vi "HFRR ADV v02.vi"() -> ()   [LabVIEW 2025] (continued)
            n3115 = local read "S 84"() -> (w4160:string)
            n3116 = local read "S 103"() -> (w4145:string)
            n3117 = local read "S 104"() -> (w4144:string)
            n3118 = property on="ENTER THE NEW PASSWORD" class="Str"("Caption.Text"=w4157) -> ()  [unwired: 2 in, 2 out]
            n3119 = property on="Password" class="Str"("Caption.Text"=w4159) -> ()  [unwired: 2 in, 2 out]
            n3120 = property on="ENTER CURRENT PASSWORD" class="Str"("Caption.Text"=w4158) -> ()  [unwired: 2 in, 2 out]
            n3121 = property on="EDIT" class="Bool (strict)"("Boolean Text.Text"=w4156) -> ()  [unwired: 2 in, 2 out]
            n3122 = property on="SAVE" class="Bool (strict)"("Boolean Text.Text"=w4160) -> ()  [unwired: 2 in, 2 out]
            n3123 = Build Array(w4145, w4144) -> (w4143:string[])
            n3124 = property on="Heater Button" class="Bool (strict)"("Strings [4]"=w4143) -> ()  [unwired: 2 in, 2 out]
            n3125 = property on="CH-HUMIDITY WET" class="DigNum (strict)"("Caption.Size to Text?"=w4146) -> ()  [unwired: 2 in, 2 out]
            n3126 = property on="CH-HUMIDITY DRY" class="DigNum (strict)"("Caption.Size to Text?"=w4146) -> ()  [unwired: 2 in, 2 out]
            n3127 = property on="CH-POWER -" class="DigNum (strict)"("Caption.Size to Text?"=w4146) -> ()  [unwired: 2 in, 2 out]
            n3128 = property on="CH-HEATER" class="DigNum (strict)"("Caption.Size to Text?"=w4146) -> ()  [unwired: 2 in, 2 out]
            n3129 = property on="CH-POWER +" class="DigNum (strict)"("Caption.Size to Text?"=w4146) -> ()  [unwired: 2 in, 2 out]
            n3130 = local read "S 92"() -> (w4155:string)
            n3131 = local read "S 93"() -> (w4154:string)
            n3132 = local read "S 105"() -> (w4141:string)
            n3133 = local read "S 106"() -> (w4140:string)
            n3134 = Build Array(w4155, w4154) -> ()  [unwired: 1 out]
            n3135 = Build Array(w4141, w4140) -> (w4142:string[])
            n3136 = local read "S 95"() -> (w4152:string)
            n3137 = local read "S 94"() -> (w4153:string)
            n3138 = local read "bs"() -> (w4168:string)
            n3139 = local read "as"() -> (w4169:string)
            n3140 = property on="Humidity" class="Bool (strict)"("Strings [4]"=w4142) -> ()  [unwired: 2 in, 2 out]
            n3141 = Concatenate Strings(w4168, "\r", w4169) -> ()  [unwired: 1 out]
            n3142 = property on="STROKE GAIN :" class="DigNum (strict)"("Caption.Text"=w4152) -> ()  [unwired: 2 in, 2 out]
            n3143 = property on="DISPLACEMENT :" class="DigNum (strict)"("Caption.Text"=w4153) -> ()  [unwired: 2 in, 2 out]
            n3144 = property on="Rh After" class="DigNum (strict)"("Caption.Size to Text?"=TRUE ("Caption.Size to Text")) -> ()  [unwired: 2 in, 2 out]
            n3145 = local read "S 48"() -> (w4192:string)
            n3146 = local read "S 50"() -> (w4190:string)
            n3147 = local read "S 51"() -> (w4189:string)
            n3148 = local read "S 49"() -> (w4191:string)
            n3149 = local read "S 52"() -> (w4188:string)
            n3150 = local read "as"() -> (w4173:string)
            n3151 = local read "bs"() -> (w4174:string)
            n3152 = local read "S 56"() -> (w4187:string)
            n3153 = local read "S 57"() -> (w4186:string)
            n3154 = local read "S 58"() -> (w4185:string)
            n3155 = local read "S 59"() -> (w4184:string)
            n3156 = property on="OPEN" class="Bool (strict)"("Boolean Text.Text"=w4188) -> ()  [unwired: 2 in, 2 out]
            n3157 = property on="OPEN 1" class="Bool (strict)"("Boolean Text.Text"=w4192) -> ()  [unwired: 2 in, 2 out]
            n3158 = property on="OPEN 2" class="Bool (strict)"("Boolean Text.Text"=w4191) -> ()  [unwired: 2 in, 2 out]
            n3159 = property on="OPEN 3" class="Bool (strict)"("Boolean Text.Text"=w4190) -> ()  [unwired: 2 in, 2 out]
            n3160 = property on="OPEN 4" class="Bool (strict)"("Boolean Text.Text"=w4189) -> ()  [unwired: 2 in, 2 out]
            n3161 = Concatenate Strings(w4174, "\r", w4173) -> ()  [unwired: 1 out]
            n3162 = local read "S 102"() -> (w4147:string)
            n3163 = property on="КОФ1" class="DigNum (strict)"("Caption.Text"=w4187) -> ()  [unwired: 2 in, 2 out]
            n3164 = local read "S 98"() -> (w4151:string)
            n3165 = local read "S 99"() -> (w4150:string)
            n3166 = local read "S 100"() -> (w4149:string)
            n3167 = local read "S 101"() -> (w4148:string)
            n3168 = property on="КОФ2" class="DigNum (strict)"("Caption.Text"=w4186) -> ()  [unwired: 2 in, 2 out]
            n3169 = property on="КОФ3" class="DigNum (strict)"("Caption.Text"=w4185) -> ()  [unwired: 2 in, 2 out]
            n3170 = property on="КОФ4" class="DigNum (strict)"("Caption.Text"=w4184) -> ()  [unwired: 2 in, 2 out]
            n3171 = local read "bs"() -> (w4172:string)
            n3172 = local read "as"() -> (w4171:string)
            n3173 = property on="CH-POWER +" class="DigNum (strict)"("Caption.Text"=w4151) -> ()  [unwired: 2 in, 2 out]
            n3174 = property on="CH-POWER -" class="DigNum (strict)"("Caption.Text"=w4150) -> ()  [unwired: 2 in, 2 out]
            n3175 = property on="CH-HEATER" class="DigNum (strict)"("Caption.Text"=w4149) -> ()  [unwired: 2 in, 2 out]
            n3176 = property on="CH-HUMIDITY DRY" class="DigNum (strict)"("Caption.Text"=w4148) -> ()  [unwired: 2 in, 2 out]
            n3177 = property on="CH-HUMIDITY WET" class="DigNum (strict)"("Caption.Text"=w4147) -> ()  [unwired: 2 in, 2 out]
            n3178 = local read "S 60"() -> (w4183:string)
            n3179 = local read "S 54"() -> (w4193:string)
            n3180 = Concatenate Strings(w4172, "\r", w4171) -> ()  [unwired: 1 out]
            n3181 = Concatenate Strings(w4193, w4183) -> ()  [unwired: 1 out]
            n3182 = local read "S 77"() -> (→"String 43":string)
            n3183 = local read "S 76"() -> (w4166:string)
            n3184 = local read "S 78"() -> (w4165:string)
            n3185 = local read "S 71"() -> (w4177:string)
            n3186 = local read "S 66"() -> (w4182:string)
            n3187 = local read "S 67"() -> (w4181:string)
            n3188 = local read "S 68"() -> (w4180:string)
            n3189 = local read "S 69"() -> (w4179:string)
            n3190 = local read "S 70"() -> (w4178:string)
            n3191 = property on="AIR TEMP" class="DigNum (strict)"("Caption.Text"=w4165) -> ()  [unwired: 2 in, 2 out]
            n3192 = property on="Set Strk" class="DigNum (strict)"("Caption.Text"=w4166) -> ()  [unwired: 2 in, 2 out]
            n3193 = property on="FRIC. FORCE :" class="DigNum (strict)"("Caption.Text"=w4182) -> ()  [unwired: 2 in, 2 out]
            n3194 = property on="TEMPERATURE :" class="DigNum (strict)"("Caption.Text"=w4181) -> ()  [unwired: 2 in, 2 out]
            n3195 = property on="SPEED OUT:" class="DigNum (strict)"("Caption.Text"=w4180) -> ()  [unwired: 2 in, 2 out]
            n3196 = property on="AIR TEMPERATURE :" class="DigNum (strict)"("Caption.Text"=w4179) -> ()  [unwired: 2 in, 2 out]
            n3197 = property on="HUMIDITY:" class="DigNum (strict)"("Caption.Text"=w4178) -> ()  [unwired: 2 in, 2 out]
            n3198 = property on="EDIT" class="Bool (strict)"("Boolean Text.Text"=w4177) -> ()  [unwired: 2 in, 2 out]
            n3199 = local read "S 79"() -> (w4164:string)
          }
          frame #2 {
          }
        }
        n3200 = local write "Lan flag"(10.0 ("Lan flag")) -> ()
      }
      frame Enabled {
      }
    }
    n3201 = Wait (ms)(milliseconds to wait=u32 2000) -> ()  [unwired: 1 out]
    n3202 = local read "Quit"() -> (w3967:bool)
  }
  n3203 = disable-structure shown="Disabled" {
    frame Disabled {
      n3204 = while {
        tunnel: [w4195] -> _
        i -> [w4195]
        stop <- w4194 continue-if-true
        n3205 = Wait (ms)(milliseconds to wait=u32 50) -> ()  [unwired: 1 out]
        n3206 = stacked-sequence {
          frame #0 {
            # "Controls Text color"
            # "Controls BG color"
            n3207 = property on="FILE" class="Str"("Text.Text Colors:Text Color"="SC  Text") -> ()  [unwired: 2 in, 2 out]
            n3208 = property on="Fuel Discription :" class="Str"("Text.Text Colors:Text Color"="SC  Text") -> ()  [unwired: 2 in, 2 out]
            n3209 = property on="tested by" class="Str"("Text.Text Colors:Text Color"="SC  Text") -> ()  [unwired: 2 in, 2 out]
            n3210 = property on="Remarks :" class="Str"("Text.Text Colors:Text Color"="SC  Text") -> ()  [unwired: 2 in, 2 out]
            n3211 = property class="DigNum (strict)"("Numeric Text.Text Colors:BG Color"="NC BG") -> ()  [unwired: 2 in, 2 out]
            n3212 = property class="DigNum (strict)"("Numeric Text.Text Colors:BG Color"="NC BG") -> ()  [unwired: 2 in, 2 out]
            n3213 = property class="DigNum (strict)"("Numeric Text.Text Colors:BG Color"="NC BG") -> ()  [unwired: 2 in, 2 out]
            n3214 = property class="DigNum (strict)"("Numeric Text.Text Colors:BG Color"="NC BG") -> ()  [unwired: 2 in, 2 out]
            n3215 = property class="DigNum (strict)"("Numeric Text.Text Colors:BG Color"="NC BG") -> ()  [unwired: 2 in, 2 out]
            n3216 = property class="DigNum (strict)"("Numeric Text.Text Colors:BG Color"="NC BG") -> ()  [unwired: 2 in, 2 out]
            n3217 = property class="DigNum (strict)"("Numeric Text.Text Colors:BG Color"="NC BG") -> ()  [unwired: 2 in, 2 out]
            n3218 = property class="DigNum (strict)"("Numeric Text.Text Colors:BG Color"="NC BG") -> ()  [unwired: 2 in, 2 out]
            n3219 = property class="DigNum (strict)"("Numeric Text.Text Colors:BG Color"="NC BG") -> ()  [unwired: 2 in, 2 out]
            n3220 = property class="DigNum (strict)"("Numeric Text.Text Colors:BG Color"="NC BG") -> ()  [unwired: 2 in, 2 out]
            n3221 = property class="DigNum (strict)"("Numeric Text.Text Colors:BG Color"="NC BG") -> ()  [unwired: 2 in, 2 out]
            n3222 = property class="DigNum (strict)"("Numeric Text.Text Colors:BG Color"="NC BG") -> ()  [unwired: 2 in, 2 out]
            n3223 = property on="FILE" class="Str"("Text.Text Colors:BG Color"="SC BG 3") -> ()  [unwired: 2 in, 2 out]
            n3224 = property on="Fuel Discription :" class="Str"("Text.Text Colors:BG Color"="SC BG 3") -> ()  [unwired: 2 in, 2 out]
            n3225 = property on="tested by" class="Str"("Text.Text Colors:BG Color"="SC BG 3") -> ()  [unwired: 2 in, 2 out]
            n3226 = property on="Remarks :" class="Str"("Text.Text Colors:BG Color"="SC BG 3") -> ()  [unwired: 2 in, 2 out]
            n3227 = property class="DigNum (strict)"("Numeric Text.Text Colors:Text Color"="NC Text") -> ()  [unwired: 2 in, 2 out]
            n3228 = property class="DigNum (strict)"("Numeric Text.Text Colors:Text Color"="NC Text") -> ()  [unwired: 2 in, 2 out]
            n3229 = property class="DigNum (strict)"("Numeric Text.Text Colors:Text Color"="NC Text") -> ()  [unwired: 2 in, 2 out]
            n3230 = property class="DigNum (strict)"("Numeric Text.Text Colors:Text Color"="NC Text") -> ()  [unwired: 2 in, 2 out]
            n3231 = property class="DigNum (strict)"("Numeric Text.Text Colors:Text Color"="NC Text") -> ()  [unwired: 2 in, 2 out]
            n3232 = property class="DigNum (strict)"("Numeric Text.Text Colors:Text Color"="NC Text") -> ()  [unwired: 2 in, 2 out]
            n3233 = property class="DigNum (strict)"("Numeric Text.Text Colors:Text Color"="NC Text") -> ()  [unwired: 2 in, 2 out]
            n3234 = property class="DigNum (strict)"("Numeric Text.Text Colors:Text Color"="NC Text") -> ()  [unwired: 2 in, 2 out]
            n3235 = property class="DigNum (strict)"("Numeric Text.Text Colors:Text Color"="NC Text") -> ()  [unwired: 2 in, 2 out]
            n3236 = property class="DigNum (strict)"("Numeric Text.Text Colors:Text Color"="NC Text") -> ()  [unwired: 2 in, 2 out]
            n3237 = property class="DigNum (strict)"("Numeric Text.Text Colors:Text Color"="NC Text") -> ()  [unwired: 2 in, 2 out]
            n3238 = property class="DigNum (strict)"("Numeric Text.Text Colors:Text Color"="NC Text") -> ()  [unwired: 2 in, 2 out]
            n3239 = property class="DigNum (strict)"("Numeric Text.Text Colors:Text Color"="NI Text  2") -> ()  [unwired: 2 in, 2 out]
            n3240 = property class="DigNum (strict)"("Numeric Text.Text Colors:Text Color"="NI Text  2") -> ()  [unwired: 2 in, 2 out]
            n3241 = property class="DigNum (strict)"("Numeric Text.Text Colors:Text Color"="NI Text  2") -> ()  [unwired: 2 in, 2 out]
            n3242 = property class="DigNum (strict)"("Numeric Text.Text Colors:Text Color"="NI Text  2") -> ()  [unwired: 2 in, 2 out]
            n3243 = property class="DigNum (strict)"("Numeric Text.Text Colors:Text Color"="NI Text  2") -> ()  [unwired: 2 in, 2 out]
            n3244 = property class="DigNum (strict)"("Numeric Text.Text Colors:Text Color"="NI Text  2") -> ()  [unwired: 2 in, 2 out]
            n3245 = property class="DigNum (strict)"("Numeric Text.Text Colors:Text Color"="NI Text  2") -> ()  [unwired: 2 in, 2 out]
            n3246 = property class="DigNum (strict)"("Numeric Text.Text Colors:Text Color"="NI Text  2") -> ()  [unwired: 2 in, 2 out]
            n3247 = property class="DigNum (strict)"("Numeric Text.Text Colors:Text Color"="NI Text  2") -> ()  [unwired: 2 in, 2 out]
            n3248 = property class="DigNum (strict)"("Numeric Text.Text Colors:Text Color"="NI Text  2") -> ()  [unwired: 2 in, 2 out]
            n3249 = property class="DigNum (strict)"("Numeric Text.Text Colors:Text Color"="NI Text  2") -> ()  [unwired: 2 in, 2 out]
            n3250 = property class="DigNum (strict)"("Numeric Text.Text Colors:Text Color"="NI Text  2") -> ()  [unwired: 2 in, 2 out]
            n3251 = property class="DigNum (strict)"("Numeric Text.Text Colors:Text Color"="NI Text  2") -> ()  [unwired: 2 in, 2 out]
            n3252 = property class="DigNum (strict)"("Numeric Text.Text Colors:Text Color"="NI Text  2") -> ()  [unwired: 2 in, 2 out]
            n3253 = property class="DigNum (strict)"("Numeric Text.Text Colors:Text Color"="NI Text  2") -> ()  [unwired: 2 in, 2 out]
            n3254 = property on="Coefficient Of Friction" class="XYGraph (strict)"("Plot Area:Colors:FG Color"="GFG  2", "Plot Area:Colors:BG Color"="GBG   2") -> ()  [unwired: 2 in, 2 out]
            n3255 = property on="Humidity ( %RH )" class="XYGraph (strict)"("Plot Area:Colors:FG Color"="GFG  2", "Plot Area:Colors:BG Color"="GBG   2") -> ()  [unwired: 2 in, 2 out]
            n3256 = property on="Air Temperature  ( °C )" class="XYGraph (strict)"("Plot Area:Colors:FG Color"="GFG  2", "Plot Area:Colors:BG Color"="GBG   2") -> ()  [unwired: 2 in, 2 out]
            n3257 = property on="Sample Temperature ( °C )" class="XYGraph (strict)"("Plot Area:Colors:FG Color"="GFG  2", "Plot Area:Colors:BG Color"="GBG   2") -> ()  [unwired: 2 in, 2 out]
            n3258 = property class="DigNum (strict)"("Numeric Text.Text Colors:BG Color"="NI BG 2") -> ()  [unwired: 2 in, 2 out]
            n3259 = property class="DigNum (strict)"("Numeric Text.Text Colors:BG Color"="NI BG 2") -> ()  [unwired: 2 in, 2 out]
            n3260 = property class="DigNum (strict)"("Numeric Text.Text Colors:BG Color"="NI BG 2") -> ()  [unwired: 2 in, 2 out]
            n3261 = property class="DigNum (strict)"("Numeric Text.Text Colors:BG Color"="NI BG 2") -> ()  [unwired: 2 in, 2 out]
            n3262 = property class="DigNum (strict)"("Numeric Text.Text Colors:BG Color"="NI BG 2") -> ()  [unwired: 2 in, 2 out]
            n3263 = property class="DigNum (strict)"("Numeric Text.Text Colors:BG Color"="NI BG 2") -> ()  [unwired: 2 in, 2 out]
            n3264 = property class="DigNum (strict)"("Numeric Text.Text Colors:BG Color"="NI BG 2") -> ()  [unwired: 2 in, 2 out]
            n3265 = property class="DigNum (strict)"("Numeric Text.Text Colors:BG Color"="NI BG 2") -> ()  [unwired: 2 in, 2 out]
            n3266 = property class="DigNum (strict)"("Numeric Text.Text Colors:BG Color"="NI BG 2") -> ()  [unwired: 2 in, 2 out]
            n3267 = property class="DigNum (strict)"("Numeric Text.Text Colors:BG Color"="NI BG 2") -> ()  [unwired: 2 in, 2 out]
            n3268 = property class="DigNum (strict)"("Numeric Text.Text Colors:BG Color"="NI BG 2") -> ()  [unwired: 2 in, 2 out]
            n3269 = property class="DigNum (strict)"("Numeric Text.Text Colors:BG Color"="NI BG 2") -> ()  [unwired: 2 in, 2 out]
            n3270 = property class="DigNum (strict)"("Numeric Text.Text Colors:BG Color"="NI BG 2") -> ()  [unwired: 2 in, 2 out]
            n3271 = property class="DigNum (strict)"("Numeric Text.Text Colors:BG Color"="NI BG 2") -> ()  [unwired: 2 in, 2 out]
            n3272 = property class="DigNum (strict)"("Numeric Text.Text Colors:BG Color"="NI BG 2") -> ()  [unwired: 2 in, 2 out]
            n3273 = property class="Bool"("Colors [4]"="Boolean BC T & BG") -> ()  [unwired: 2 in, 2 out]
            n3274 = property on="Save & Continue" class="Bool (strict)"("Colors [4]"="Boolean BC T & BG") -> ()  [unwired: 2 in, 2 out]
            n3275 = property on="Heater Button" class="Bool (strict)"("Colors [4]"="Boolean BC T & BG") -> ()  [unwired: 2 in, 2 out]
            n3276 = property class="Bool"("Colors [4]"="Boolean BC T & BG") -> ()  [unwired: 2 in, 2 out]
            n3277 = property on="Humidity" class="Bool (strict)"("Colors [4]"="Boolean BC T & BG") -> ()  [unwired: 2 in, 2 out]
            n3278 = property class="Bool (strict)"("Colors [4]"="Boolean BC T & BG") -> ()  [unwired: 2 in, 2 out]
            n3279 = property on="RUN" class="Bool (strict)"("Colors [4]"="Boolean BC T & BG") -> ()  [unwired: 2 in, 2 out]
            n3280 = property on="trip1 8" class="Bool (strict)"("Colors [4]"="Boolean BC T & BG") -> ()  [unwired: 2 in, 2 out]
            n3281 = property class="Bool"("Colors [4]"="Boolean BC T & BG") -> ()  [unwired: 2 in, 2 out]
            n3282 = property class="Bool (strict)"("Colors [4]"="Boolean BC T & BG") -> ()  [unwired: 2 in, 2 out]
            n3283 = property on="OPEN 1" class="Bool (strict)"("Colors [4]"="Boolean BC T & BG 2") -> ()  [unwired: 2 in, 2 out]
            n3284 = property on="OPEN 2" class="Bool (strict)"("Colors [4]"="Boolean BC T & BG 2") -> ()  [unwired: 2 in, 2 out]
            n3285 = property on="OPEN 3" class="Bool (strict)"("Colors [4]"="Boolean BC T & BG 2") -> ()  [unwired: 2 in, 2 out]
            n3286 = property on="OPEN 4" class="Bool (strict)"("Colors [4]"="Boolean BC T & BG 2") -> ()  [unwired: 2 in, 2 out]
            n3287 = property on="OPEN" class="Bool (strict)"("Colors [4]"="Boolean BC T & BG 2") -> ()  [unwired: 2 in, 2 out]
            n3288 = property on="rstv2" class="Bool"("Colors [4]"="Boolean BC T & BG 2") -> ()  [unwired: 2 in, 2 out]
            n3289 = property on="RST CP" class="Bool"("Colors [4]"="Boolean BC T & BG 2") -> ()  [unwired: 2 in, 2 out]
            n3290 = property on="RSTV1 3" class="Bool"("Colors [4]"="Boolean BC T & BG 2") -> ()  [unwired: 2 in, 2 out]
            n3291 = property on="RSTV1 2" class="Bool"("Colors [4]"="Boolean BC T & BG 2") -> ()  [unwired: 2 in, 2 out]
          }
          frame #1 {
          }
        }
        n3292 = local read "Quit"() -> (w4194:bool)
      }
    }
    frame Enabled {
    }
  }
  n3293 = while {
    shift-right: [w4212] -> _
    shift-left: _ -> [w4213]
    shift-right: [w4210] -> _
    shift-left: T14 {"Read Heave and Surge"="", "Bytes at Heave Port"=0.0, "Heave and Surge COM Port:"="COM9", "Com Port 2"="COM7", "Residual Due"="", "Heave COM Status 2"=TRUE, "Heave COM Status"=TRUE, "Port 2"=TRUE, "Sway PPR"=6400.0, "Surge PPR"=6400.0, "Heave PPR"=6400.0, "Sway Pitch"=2.0, "Surge Pitch"=3.0, "Heave Pitch"=4.0, "Sway Pulses/mm"=320.0, "Surge Pulses/mm"=1600.0, "Heave Pulses/mm"=1600.0, "inner loop"=0.0, "Read Heave and Surge 2"="", "String 36"="", "Write S"=FALSE, "WriteCC1"=[""], "Heave COM Loop"=0, "LastCom"="", "EXIT"=FALSE, "Error Heave"={"status"=TRUE, "code"=-1073807343, "source"=""}} -> [w4209]
    shift-right: [w4207] -> _
    shift-left: enum16{"init", "MAIN", "Panel Close"}."init" -> [w4208]
    stop <- w4211 stop-if-true
    n3294 = case shown="\"init\"" w4208 {
      tunnel: w4213 -> [w4227 w4242 w4312 w4314]
      tunnel: [w4221 w4260 w4312 w4314] -> w4212
      tunnel: [_ _ TRUE _] -> w4211
      tunnel: [w4217 w4257 w4310 w4313] -> w4210
      tunnel: w4209 -> [w4224 w4241 w4310 w4313]
      tunnel: [enum16{"init", "MAIN", "Panel Close"}."MAIN" w4235 _ _] -> w4207
      frame "init" {
        n3295 = Bundle By Name(cluster=w4224, "Heave and Surge COM Port:"="C3 :") -> (w4223:T14)
        n3296 = call "Instrument fgv.vi"("Enum"=T24."INIT", "error in (no error) 2"=w4227, "INPUT"=w4223) -> ("error"=w4225:errorcluster, "output"=w4220:T14)  [unwired: 6 in, 1 out]
        n3297 = case shown="No Error" w4225 {
          selector: w4225 -> [w4229 _]
          tunnel: [w4229 w4233] -> w4221
          tunnel: w4220 -> [w4228 w4231]
          tunnel: [w4228 w4230] -> w4218
          frame No Error {
          }
          frame Error {
            n3298 = call "Instrument fgv.vi"("Enum"=T24."ERROR INIT", "INPUT"=w4231) -> ("error"=w4234:errorcluster, "output"=w4230:T14)  [unwired: 7 in, 1 out]
            n3299 = call <vilib>:"Clear Errors.vi"("error in (no error)"=w4234) -> ("error out"=w4233:errorcluster)  [unwired: 5 in, 1 out]
          }
        }
        n3300 = local read "LastCom"() -> (w4216:string)
        n3301 = Unbundle By Name(w4218) -> ("Heave COM Status 2"=→"COM Status" →"Instrument Status":bool, "Error Heave"=→"Error":errorcluster)  [unwired: 1 out]
        n3302 = Bundle By Name(cluster=w4218, "LastCom"=w4216) -> (w4217:T14)
      }
      frame "MAIN" {
        n3303 = Unbundle By Name(w4241) -> ("Com Port 2"=w4262:refnum<visa-resource-name>)
        n3304 = local write "Com Port 4"(w4262) -> ()
        n3305 = local read "C3 :"() -> (w4239:refnum<visa-resource-name>)
        n3306 = Divide(x="Heave PPR", y="Heave Pitch") -> (x/y=→"Heave Pulses/mm":dbl)
        n3307 = Bundle By Name(cluster=w4241, "Heave and Surge COM Port:"=w4239) -> (w4240:T14)
        n3308 = Equal?(x=w4262, y=w4239) -> (x = y?=w4261:bool)
        n3309 = Divide(x="Sway PPR", y="Sway Pitch") -> (x/y=→"Sway Pulses/mm":dbl)
        n3310 = case shown="False" w4261 {
          tunnel: [w4266 w4283] -> w4260
          tunnel: w4242 -> [w4267 w4289]
          tunnel: w4240 -> [w4265 w4287]
          tunnel: [w4264 w4282] -> w4257
          frame False {
            n3311 = call <vilib>:"Clear Errors.vi"("error in (no error)"=w4267) -> ("error out"=w4263:errorcluster)  [unwired: 5 in, 1 out]
            n3312 = call "Instrument fgv.vi"("Enum"=T24."ERROR INIT", "error in (no error) 2"=w4263, "INPUT"=w4265) -> ("error"=w4269:errorcluster, "output"=w4264:T14)  [unwired: 6 in, 1 out]
            n3313 = call <vilib>:"Clear Errors.vi"("error in (no error)"=w4269) -> ("error out"=w4266:errorcluster)  [unwired: 5 in, 1 out]
          }
          frame True {
            n3314 = call "Instrument fgv.vi"("Enum"=T24."READ", "error in (no error) 2"=w4289, "INPUT"=w4287) -> ("error"=w4288:errorcluster, "output"=w4279:T14)  [unwired: 6 in, 1 out]
            n3315 = Bundle By Name(cluster=w4279, "String 36"="String 11") -> (w4278:T14)
            n3316 = case shown="True" "Write S" {
              selector: "Write S" -> [_ w4309]
              tunnel: w4288 -> [w4302 w4308]
              tunnel: [w4302 w4307] -> w4275
              tunnel: w4278 -> [w4301 w4304]
              tunnel: [w4301 w4303] -> w4274
              frame False {
              }
              frame True {
                n3317 = Not(x=w4309) -> (.not. x?=w4305:bool)
                n3318 = local write "Write S"(w4305) -> ()
                n3319 = call "Instrument fgv.vi"("Enum"=T24."MANUAL WRITE", "error in (no error) 2"=w4308, "INPUT"=w4304) -> ("error"=w4307:errorcluster, "output"=w4303:T14)  [unwired: 6 in, 1 out]
              }
            }
            n3320 = Array Size(array="WriteHumidity") -> (size(s)=w4272:i32)
            n3321 = Greater Than 0?(x=w4272) -> (x > 0?=w4270:bool)
            n3322 = call "Instrument fgv.vi"("Enum"=T24."WRITE", "error in (no error) 2"=w4275, "WriteCC1"="WriteHumidity", "INPUT"=w4274) -> ("error"=w4285:errorcluster, "WriteCC1 2"=w4273:string[], "output"=w4284:T14)  [unwired: 5 in]
            n3323 = case shown="True" w4270 {
              tunnel: w4273 -> [_ w4291]
              frame False {
              }
              frame True {
                n3324 = local write "WriteHumidity"(w4291) -> ()
              }
            }
            n3325 = case shown="Error" w4285 {
              selector: w4285 -> [w4292 w4295]
              tunnel: w4284 -> [w4293 w4300]
              tunnel: [w4293 w4299] -> w4282
              tunnel: [w4292 w4297] -> w4283
              frame No Error {
              }
              frame Error {
                n3326 = call <vilib>:"Clear Errors.vi"("error in (no error)"=w4295) -> ("error out"=w4294:errorcluster)  [unwired: 5 in, 1 out]
                n3327 = call "Instrument fgv.vi"("Enum"=T24."ERROR INIT", "error in (no error) 2"=w4294, "INPUT"=w4300) -> ("error"=w4298:errorcluster, "output"=w4299:T14)  [unwired: 6 in, 1 out]
                n3328 = call <vilib>:"Clear Errors.vi"("error in (no error)"=w4298) -> ("error out"=w4297:errorcluster)  [unwired: 5 in, 1 out]
              }
            }
            n3329 = Unbundle By Name(w4282) -> ("LastCom"=→"LastCom":string, "Read Heave and Surge"=→"Read Humidity":string)
          }
        }
        n3330 = Divide(x="Surge PPR", y="Surge Pitch") -> (x/y=→"Surge Pulses/mm":dbl)
        n3331 = Unbundle By Name(w4257) -> ("Heave COM Status 2"=w4259:bool, "Heave COM Status"=w4258:bool, "Error Heave"=w4255:errorcluster, "Bytes at Heave Port"=→"Bytes at Humidity Port":dbl)
        n3332 = Unbundle By Name(w4255) -> ("status"=→"Humidity Port":bool)
        n3333 = Not(x=w4258) -> (.not. x?=w4243:bool)
        n3334 = local write "Error"(w4255) -> ()
        n3335 = Not(x=w4259) -> (.not. x?=w4244:bool)
        n3336 = local write "Instrument Status"(w4243) -> ()
        n3337 = local write "COM Status"(w4244) -> ()
        n3338 = local read "Quit"() -> (w4236:bool)
        n3339 = Select(t=enum16{"init", "MAIN", "Panel Close"}."Panel Close", s=w4236, f=enum16{"init", "MAIN", "Panel Close"}."MAIN") -> (s? t:f=w4235:enum16{"init", "MAIN", "Panel Close"})
      }
      frame "Panel Close" {
      }
      frame Default {
      }
    }
  }
  n3340 = while {
    stop <- w4340 stop-if-true
    n3341 = local read "Read Humidity"() -> (w4321:string)
    n3342 = call <vilib>:"High Resolution Polling Wait.vi"("seconds to wait"=0.1) -> ()  [unwired: 10 in, 1 out]
    n3343 = Spreadsheet String To Array(delimiter (Tab)=",", format string="", spreadsheet string=w4321, array type (2D Dbl)=string[] []) -> (array=w4335:string[])
    n3344 = for {
      tunnel: w4335 -> [w4345] mode=indexing
      tunnel: string[] ["STATE;", "SET;", "RH;", "T;", "AMB_RH;", "AMB_T;", "PUMP;", "FAN_IN;", "FAN_OUT;", "DEHUM;", "CURRENT;", "STALL;"] -> [w4344] mode=indexing
      tunnel: [w4343] -> w4334 mode=indexing
      n3345 = Match Pattern(string=w4345, regular expression=w4344) -> (after substring=w4343:string)  [unwired: 1 in, 3 out]
    }
    n3346 = Index Array(array=w4334) -> (element #1=→"STATE :":string, element #2=→"SET :":string, element #3=w4323:string, element #4=→"T :":string, element #5=w4320:string, element #6=→"AMB_T :":string, element #7=→"PUMP :":string, element #8=→"FAN_IN :":string, element #9=→"FAN_OUT :":string, element #10=→"DEHUM :":string, element #11=→"CURRENT :":string, element #12=→"STALL :":string)  [unwired: 12 in]
    "RH :" <- w4323
    "AMB_RH :" <- w4320
    n3347 = Fract/Exp String To Number(string=w4323) -> (number=w4315:dbl)  [unwired: 3 in, 1 out]
    n3348 = Fract/Exp String To Number(string=w4320) -> (number=w4319:dbl)  [unwired: 3 in, 1 out]
    n3349 = local write "Ambient Humidity :"(w4319) -> ()
    n3350 = Equal?(x=w4315, y=0.0) -> (x = y?=w4317:bool)
    n3351 = case shown="True" w4317 {
      tunnel: [w4341 w4342] -> w4316
      tunnel: w4315 -> [w4341 _]
      frame False {
        (unwired) 0.0
        "Humidity temp" <- w4341
      }
      frame True {
        n3352 = local read "Humidity temp"() -> (w4342:dbl)
      }
    }
    "RH Numeric:" <- w4316
    n3353 = local read "Quit"() -> (w4340:bool)
  }
  n3354 = disable-structure shown="Disabled" {
    frame Disabled {
      n3355 = while {
        tunnel: [w4579] -> _
        i -> [w4579]
        stop <- w4576 stop-if-true
        n3356 = local read "powstat"() -> (w4577:bool)
        n3357 = case shown="True" w4577 {
          frame False {
          }
          frame True {
            n3358 = local read "RUN"() -> (w4580:bool)
            n3359 = case shown="True" w4580 {
              frame False {
                w4610 = 65.0 ("y")
                n3360 = local read "Set Hz"() -> (w4638:dbl)
                n3361 = local read "NORMAL LOAD"() -> (w4639:dbl)
                n3362 = Multiply(x=w4638, y=60.0) -> (x*y=w4645:dbl)
                n3363 = Multiply(x=1.2 ("y"), y=0.949) -> (x*y=w4614:dbl)
                n3364 = Multiply(x=1.2 ("y"), y=0.8166) -> (x*y=w4618:dbl)
                n3365 = Multiply(x=1.2 ("y"), y=0.851) -> (x*y=w4613:dbl)
                n3366 = local read "FF 2"() -> (w4637:dbl)
                n3367 = Absolute Value(x=w4645) -> (abs(x)=w4643:dbl)
                n3368 = case shown="13.." w4637 {
                  tunnel: [1 2 3] -> w4635
                  frame 0..10, Default {
                    # "Normal"
                  }
                  frame 11, 12 {
                  }
                  frame 13.. {
                  }
                }
                "FF STATE" <- w4635
                n3369 = local read "TEMP"() -> (w4598:dbl)
                n3370 = local read item#-1() -> (w4612)
                n3371 = Less?(x=w4612, y=w4618) -> (x < y?=w4615:bool)
                n3372 = In Range and Coerce(upper limit=w4614, x=w4612, lower limit=w4613) -> (In Range?=w4616:bool)  [unwired: 1 out]
                n3373 = case shown="3601.." w4643 {
                  tunnel: [1 2 3] -> w4641
                  frame 0..3000, Default {
                    # "Normal"
                  }
                  frame 3001..3600 {
                  }
                  frame 3601.. {
                  }
                }
                n3374 = case shown="11.." w4639 {
                  tunnel: [1 3] -> w4640
                  frame 1..10, Default {
                  }
                  frame 11.. {
                  }
                }
                "NL STATE" <- w4640
                n3375 = Multiply(x=1.2 ("y"), y=0.95) -> (x*y=w4628:dbl)
                n3376 = Multiply(x=w4610, y=0.954) -> (x*y=w4602:dbl)
                n3377 = Or(x=w4615, y=w4616) -> (x .or. y?=w4617:bool)
                n3378 = Greater Or Equal?(x=w4612, y=w4628) -> (x >= y?=w4625:bool)
                n3379 = Multiply(x=w4610, y=0.99) -> (x*y=w4599:dbl)
                n3380 = Greater Or Equal?(x=w4598, y=w4599) -> (x >= y?=w4604:bool)
                n3381 = Greater Or Equal?(x=w4598, y=w4602) -> (x >= y?=w4601:bool)
                n3382 = case shown="0, 1, Default" w4612 {
                  tunnel: [1 3] -> w4629
                  frame 0, 1, Default {
                  }
                  frame 2.. {
                  }
                }
                n3383 = case shown="True" w4625 {
                  tunnel: [1 3] -> w4630
                  frame False {
                  }
                  frame True {
                  }
                }
                n3384 = case shown="True" w4617 {
                  tunnel: [1 2] -> w4631
                  frame False {
                  }
                  frame True {
                  }
                }
                n3385 = case shown="..0" w4598 {
                  tunnel: [2 3 3 1] -> w4605
                  frame 61, 62 {
                  }
                  frame 63.. {
                  }
                  frame ..0 {
                  }
                  frame 10..60, Default {
                  }
                }
                n3386 = case shown="True" w4604 {
                  tunnel: [1 3] -> w4606
                  frame False {
                  }
                  frame True {
                  }
                }
                n3387 = Number To Decimal String(number=w4641) -> (decimal integer string=w4642:string)  [unwired: 1 in]
                n3388 = case shown="True" w4601 {
                  tunnel: [1 2] -> w4607
                  frame False {
                  }
                  frame True {
                  }
                }
                n3389 = Number To Decimal String(number=1) -> (decimal integer string=→"Air temp":string)  [unwired: 1 in]
                n3390 = Number To Decimal String(number=w4635) -> (decimal integer string=→"ff_st":string)  [unwired: 1 in]
                n3391 = local write "sp_st"(w4642) -> ()
                n3392 = Number To Decimal String(number=w4640) -> (decimal integer string=→"nl_st":string)  [unwired: 1 in]
                n3393 = Build Array(w4605, w4606, w4607) -> (w4608:i32[])
                n3394 = Build Array(w4629, w4630, w4631) -> (w4632:i32[])
                n3395 = Array Max & Min(array=w4608) -> (max value=w4609:i32)  [unwired: 3 out]
                n3396 = Array Max & Min(array=w4632) -> (max value=w4633:i32)  [unwired: 3 out]
                n3397 = Number To Decimal String(number=w4609) -> (decimal integer string=w4597:string)  [unwired: 1 in]
                n3398 = Number To Decimal String(number=w4633) -> (decimal integer string=→"Stroke Ln 2":string)  [unwired: 1 in]
                n3399 = local write "temp_st"(w4597) -> ()
              }
              frame True {
                w4695 = 65.0 ("y")
                # "Healthy -1\nWarning -2\nError -3"
                n3400 = local read "TEMP"() -> (w4706:dbl)
                n3401 = local read "NORMAL LOAD"() -> (w4710:dbl)
                n3402 = local read "Set Hz"() -> (w4708:dbl)
                n3403 = Multiply(x=1.2 ("y"), y=0.949) -> (x*y=w4690:dbl)
                n3404 = Multiply(x=1.2 ("y"), y=0.8166) -> (x*y=w4686:dbl)
                n3405 = Multiply(x=1.2 ("y"), y=0.851) -> (x*y=w4691:dbl)
                n3406 = Multiply(x=w4695, y=0.954) -> (x*y=w4702:dbl)
                n3407 = Multiply(x=w4695, y=0.99) -> (x*y=w4705:dbl)
                n3408 = Greater Or Equal?(x=w4706, y=w4705) -> (x >= y?=w4700:bool)
                n3409 = Multiply(x=w4708, y=60.0) -> (x*y=w4714:dbl)
                n3410 = Greater Or Equal?(x=w4706, y=w4702) -> (x >= y?=w4703:bool)
                n3411 = local read "FF 2"() -> (w4709:dbl)
                n3412 = local read item#-1() -> (w4692)
                n3413 = Less?(x=w4692, y=w4686) -> (x < y?=w4689:bool)
                n3414 = In Range and Coerce(upper limit=w4690, x=w4692, lower limit=w4691) -> (In Range?=w4688:bool)  [unwired: 1 out]
                n3415 = Absolute Value(x=w4714) -> (abs(x)=w4712:dbl)
                n3416 = case shown="63.." w4706 {
                  tunnel: [2 3 3 1] -> w4699
                  frame 61, 62 {
                  }
                  frame 63.. {
                  }
                  frame ..0 {
                  }
                  frame 10..60, Default {
                  }
                }
                n3417 = case shown="True" w4700 {
                  tunnel: [1 3] -> w4698
                  frame False {
                  }
                  frame True {
                  }
                }
                n3418 = case shown="True" w4703 {
                  tunnel: [1 2] -> w4697
                  frame False {
                  }
                  frame True {
                  }
                }
                n3419 = Multiply(x=1.2 ("y"), y=0.95) -> (x*y=w4676:dbl)
                n3420 = case shown="1..10, Default" w4710 {
                  tunnel: [1 3] -> w4717
                  frame 1..10, Default {
                  }
                  frame 11.. {
                  }
                }
                n3421 = case shown="0..10, Default" w4709 {
                  tunnel: [1 2 3] -> w4716
                  frame 0..10, Default {
                  }
                  frame 11, 12 {
                  }
                  frame 13.. {
                  }
                }
                n3422 = case shown="3601.." w4712 {
                  tunnel: [1 2 3] -> w4711
                  frame 0..3000, Default {
                    # "Normal"
                  }
                  frame 3001..3600 {
                  }
                  frame 3601.. {
                  }
                }
                n3423 = Or(x=w4689, y=w4688) -> (x .or. y?=w4687:bool)
                n3424 = Greater Or Equal?(x=w4692, y=w4676) -> (x >= y?=w4679:bool)
                n3425 = case shown="0, 1, Default" w4692 {
                  tunnel: [1 3] -> w4675
                  frame 0, 1, Default {
                  }
                  frame 2.. {
                  }
                }
                n3426 = case shown="True" w4679 {
                  tunnel: [1 3] -> w4674
                  frame False {
                  }
                  frame True {
                  }
                }
                n3427 = case shown="True" w4687 {
                  tunnel: [1 2] -> w4673
                  frame False {
                  }
                  frame True {
                  }
                }
                n3428 = Build Array(w4699, w4698, w4697) -> (w4696:i32[])
                n3429 = Number To Decimal String(number=w4711) -> (decimal integer string=→"sp_st":string)  [unwired: 1 in]
                n3430 = Array Max & Min(array=w4696) -> (max value=w4693:i32)  [unwired: 3 out]
                "TEMP STATE" <- w4693
                n3431 = Number To Decimal String(number=w4717) -> (decimal integer string=w4720:string)  [unwired: 1 in]
                n3432 = Number To Decimal String(number=w4716) -> (decimal integer string=w4718:string)  [unwired: 1 in]
                n3433 = Number To Decimal String(number=w4693) -> (decimal integer string=→"temp_st":string)  [unwired: 1 in]
                n3434 = Build Array(w4675, w4674, w4673) -> (w4672:i32[])
                n3435 = local write "nl_st"(w4720) -> ()
                n3436 = local write "ff_st"(w4718) -> ()
                n3437 = Number To Decimal String(number=1) -> (decimal integer string=w4715:string)  [unwired: 1 in]
                n3438 = Array Max & Min(array=w4672) -> (max value=w4671:i32)  [unwired: 3 out]
                n3439 = local write "Air temp"(w4715) -> ()
                n3440 = Number To Decimal String(number=w4671) -> (decimal integer string=w4670:string)  [unwired: 1 in]
                n3441 = local write "Stroke Ln 2"(w4670) -> ()
              }
            }
            n3442 = local read "Stroke Ln 2"() -> (w4582:string)
            n3443 = local read "nl_st"() -> (w4588:string)
            n3444 = local read "ff_st"() -> (w4585:string)
            n3445 = local read "sp_st"() -> (w4586:string)
            n3446 = local read "temp_st"() -> (w4587:string)
            n3447 = local read "Air temp"() -> (w4581:string)
            n3448 = Replace Array Subset(array="in", new element #1=w4588, index #1=1 ("index"), new element #2=w4585, index #2=2 ("index"), new element #3=w4587, index #3=3 ("index"), new element #4=w4586, index #4=4 ("index"), new element #5=w4582, index #5=5 ("index"), new element #6=w4581, index #6=6 ("index"), new element #7="Sensor State" ("new element/subarray"), index #7=0 ("index")) -> (→"out":string[])
          }
        }
        n3449 = Wait (ms)(milliseconds to wait=u32 10) -> ()  [unwired: 1 out]
        n3450 = local read "Quit"() -> (w4576:bool)
      }
      n3451 = while {
        stop <- w4551 stop-if-true
        n3452 = local read "run replace"() -> (w4553:bool)
        n3453 = Wait (ms)(milliseconds to wait=u32 100) -> ()  [unwired: 1 out]
        n3454 = Equal?(x="FLAG 2", y=0.0) -> (x = y?=w4554:bool)
        n3455 = case shown="True" w4554 {
          frame False {
          }
          frame True {
            n3456 = local write "FLAG 2"(100.0 ("FLAG 2")) -> ()
            n3457 = call <vilib>:"Read Characters From File.vi"("file path (dialog if empty)"=path "C:/LAB-IQ-NXT/WO 2449 TT.sig", "convert eol? (no:F)"=FALSE ("append to file? (new file:F)")) -> ("character string"=w4557:string)  [unwired: 4 in, 3 out]
            n3458 = call <vilib>:"Read Characters From File.vi"("file path (dialog if empty)"=path "C:/LAB-IQ-NXT/WO 2449 TRH.sig", "convert eol? (no:F)"=FALSE ("append to file? (new file:F)")) -> ("character string"=w4558:string)  [unwired: 4 in, 3 out]
            n3459 = Decimal String To Number(string=w4557) -> (number=w4559:i32)  [unwired: 2 in, 1 out]
            n3460 = local write "Total No. of Tests"(w4559) -> ()
            n3461 = Decimal String To Number(string=w4558) -> (number=w4562:i32)  [unwired: 2 in, 1 out]
            n3462 = local write "SEN.RUN HRS"(w4562) -> ()
          }
        }
        n3463 = case shown="True" w4553 {
          frame False {
          }
          frame True {
            n3464 = Equal?(x="FLAG 4", y=0.0) -> (x = y?=w4566:bool)
            n3465 = case shown="False" w4566 {
              frame False {
                n3466 = Get Date/Time In Seconds() -> (seconds since 1Jan1904=w4572:timestamp)
                n3467 = local read "START 3"() -> (w4570:dbl)
                n3468 = To Double Precision Float(number=w4572) -> (double precision float=w4571:dbl)
                n3469 = Subtract(x=w4571, y=w4570) -> (x-y=→"SENSOR TIME":dbl)
              }
              frame True {
                n3470 = Get Date/Time In Seconds() -> (seconds since 1Jan1904=w4574:timestamp)
                n3471 = local write "FLAG 4"(100.0 ("FLAG")) -> ()
                n3472 = To Double Precision Float(number=w4574) -> (double precision float=→"START 3":dbl)
              }
            }
          }
        }
        n3473 = local read "Quit"() -> (w4551:bool)
      }
      n3474 = while {
        shift-right: [w4351] -> _
        shift-left: _ -> [w4352]
        tunnel: [w4347] -> _
        i -> [w4347]
        stop <- w4346 stop-if-true
        n3475 = Wait (ms)(milliseconds to wait=u32 50 ("Refresh Rate (ms)")) -> ()  [unwired: 1 out]
        n3476 = local read "Json End Flg"() -> (w4348:bool)
        n3477 = Not(x="Upld AR 2") -> ()  [unwired: 1 out]
        n3478 = local read "Upld AR 2"() -> (w4349:bool)
        n3479 = call "Elapsed Time9"("Time Target (s)"="Sen.Upload Rate (s)", "Reset"=FALSE, "Auto Reset"=TRUE) -> ("Time has Elapsed"=w4358:bool)  [unwired: 9 in, 7 out]
        n3480 = Or(x=w4358, y=w4348) -> (x .or. y?=w4354:bool)
        n3481 = case shown="True" w4354 {
          frame False {
          }
          frame True {
            w4450 = "\"SensorName\":\"" ("string")
            w4420 = " \"},{"
            w4445 = "\",\"SensorState\":\""
            w4447 = "\",\"SensorModelNumber\":\"" ("string")
            w4446 = "\",\"SensorRuntimeHours\":\"" ("string")
            n3482 = local read "model num"() -> (w4444:string[])
            n3483 = local read "Sensor name"() -> (w4463:string[])
            n3484 = local read "run"() -> (w4434:string[])
            n3485 = local read "SENSOR TIME"() -> (w4390:dbl)
            n3486 = local read "out"() -> (w4383:string[])
            n3487 = local read "Total No. of Tests"() -> (w4388:dbl)
            n3488 = Select(t=60.0, s="Run test 3", f=3600.0) -> (s? t:f=w4398:dbl)
            n3489 = Index Array(array=w4444, index #1=1 ("index")) -> (element #1=w4443:string, element #2=w4442:string, element #3=w4441:string, element #4=w4440:string, element #5=w4439:string, element #6=w4438:string)  [unwired: 5 in]
            n3490 = Index Array(array=w4434, index #1=1 ("index")) -> (element #1=w4433:string, element #2=w4432:string, element #3=w4431:string, element #4=w4430:string, element #5=w4429:string, element #6=w4428:string)  [unwired: 5 in]
            n3491 = Index Array(array=w4463, index #1=1 ("index")) -> (element #1=w4462:string, element #2=w4461:string, element #3=w4460:string, element #4=w4459:string, element #5=w4449:string, element #6=w4448:string)  [unwired: 5 in]
            n3492 = Index Array(array=w4383, index #1=1 ("index")) -> (element #1=w4415:string, element #2=w4414:string, element #3=w4413:string, element #4=w4412:string, element #5=w4411:string, element #6=w4410:string)  [unwired: 5 in]
            n3493 = local read "SEN.RUN HRS"() -> (w4386:dbl)
            n3494 = Divide(x=w4390, y=w4398) -> (x/y=w4397:dbl)
            n3495 = Increment(x=w4397) -> (x+1=w4393:dbl)
            n3496 = Number To Decimal String(number=w4393) -> (decimal integer string=→"run hrs":string)  [unwired: 1 in]
            n3497 = Divide(x=w4386, y=3600.0 ("f")) -> (x/y=w4381:dbl)
            n3498 = Round To Nearest(number=w4381) -> (nearest integer value=w4379:dbl)
            n3499 = Number To Decimal String(number=w4379) -> (decimal integer string=w4380:string)  [unwired: 1 in]
            n3500 = Number To Decimal String(number=w4388) -> (decimal integer string=w4389:string)  [unwired: 1 in]
            n3501 = local read "Model No"() -> (w4394:string)
            n3502 = local read "UUID"() -> (w4489:string)
            n3503 = local read "Serial No"() -> (w4493:string)
            n3504 = local read "Secret Key"() -> (w4494:string)
            n3505 = Concatenate Strings("\",\"MachineSerialNumber\":\"" ("string"), w4493) -> (w4497:string)
            n3506 = Concatenate Strings("\",\"ModelNumber\":\"" ("string"), w4394) -> (w4395:string)
            n3507 = Concatenate Strings("\",\"MachineRuntimeHours\":\"" ("string"), w4380) -> (w4498:string)
            n3508 = Concatenate Strings("\",\"MachineRuntimeCycles\":\"", w4389) -> (w4491:string)
            n3509 = Concatenate Strings(w4447, w4443) -> (w4477:string)
            n3510 = Concatenate Strings(w4446, w4433) -> (w4478:string)
            n3511 = Concatenate Strings(w4445, w4415) -> (w4476:string)
            n3512 = Concatenate Strings(w4497, w4395, w4498, w4491) -> (w4500:string)
            n3513 = Concatenate Strings(w4447, w4442) -> (w4474:string)
            n3514 = Concatenate Strings(w4446, w4432) -> (w4473:string)
            n3515 = Concatenate Strings(w4445, w4414) -> (w4475:string)
            n3516 = Concatenate Strings(w4447, w4441) -> (w4469:string)
            n3517 = Concatenate Strings(w4446, w4431) -> (w4470:string)
            n3518 = Concatenate Strings(w4445, w4413) -> (w4468:string)
            n3519 = Concatenate Strings(w4447, w4440) -> (w4466:string)
            n3520 = Concatenate Strings(w4446, w4430) -> (w4465:string)
            n3521 = Concatenate Strings(w4445, w4412) -> (w4467:string)
            n3522 = Concatenate Strings(w4477, w4478, w4476) -> (w4479:string)
            n3523 = Concatenate Strings(w4447, w4439) -> (w4456:string)
            n3524 = Concatenate Strings(w4446, w4429) -> (w4457:string)
            n3525 = Concatenate Strings(w4447, w4438) -> (w4453:string)
            n3526 = Concatenate Strings(w4446, w4428) -> (w4452:string)
            n3527 = Concatenate Strings(w4445, w4411) -> (w4455:string)
            n3528 = Concatenate Strings(w4445, w4410) -> (w4454:string)
            n3529 = Concatenate Strings("{\"SecretKey\":\"", w4494, w4500, "\",\"UUID\" : \"", w4489, "\",\"SensorInformation\":", "[{" ("string")) -> (w4427:string)
            n3530 = Concatenate Strings(w4474, w4473, w4475) -> (w4472:string)
            n3531 = Concatenate Strings(w4469, w4470, w4468) -> (w4471:string)
            n3532 = Concatenate Strings(w4466, w4465, w4467) -> (w4464:string)
            n3533 = Concatenate Strings(w4456, w4457, w4455) -> (w4458:string)
            n3534 = Concatenate Strings(w4453, w4452, w4454) -> (w4451:string)
            n3535 = Concatenate Strings(w4450, w4462, w4479, w4420) -> (w4426:string)
            n3536 = Concatenate Strings(w4450, w4461, w4472, w4420) -> (w4425:string)
            n3537 = Concatenate Strings(w4450, w4460, w4471, w4420) -> (w4424:string)
            n3538 = Concatenate Strings(w4450, w4459, w4464, w4420) -> (w4423:string)
            n3539 = Concatenate Strings(w4450, w4449, w4458, w4420) -> (w4422:string)
            n3540 = Concatenate Strings(w4450, w4448, w4451, "\"}" ("string")) -> (w4421:string)
            n3541 = Concatenate Strings(w4427, w4426, w4425, w4424, w4423, w4422, w4421, "]}" ("string")) -> (w4418:string)
            n3542 = local read "SEN.RUN HRS"() -> (w4385:dbl)
            n3543 = disable-structure shown="Disabled" {
              frame Disabled {
                n3544 = local read "state"() -> (w4504:string[])
                n3545 = Delete From Array(array=w4504, index=0) -> (array with subset deleted=w4502:string[])  [unwired: 1 in, 1 out]
                n3546 = for {
                  N: 6 -> [_]
                  tunnel: w4502 -> [w4515] mode=indexing
                  tunnel: [w4514] -> w4501 mode=indexing
                  n3547 = Equal?(x=w4515, y="Warning") -> (x = y?=w4511:bool)
                  n3548 = Equal?(x=w4515, y="Healthy") -> (x = y?=w4508:bool)
                  n3549 = Select(t="2" ("y"), s=w4511, f="3" ("y")) -> (s? t:f=w4506:string)
                  n3550 = Select(t="1" ("y"), s=w4508, f=w4506) -> (s? t:f=w4514:string)
                }
                "state1" <- w4501
              }
              frame Enabled {
              }
            }
            n3551 = stacked-sequence {
              tunnel: w4418 -> [w4526 _ _]
              tunnel: [_ _ w4542] -> _
              frame #0 {
                (unwired) FALSE ("convert eol (F)")
                w4528 = enum16{"start", "end", "current"}."start" ("pos mode (0:2)")
                n3552 = local read "Path"() -> (w4522:path)
                n3553 = Path To String(path=w4522) -> (string=w4534:string)
                n3554 = Concatenate Strings(w4534, "\\", "Sensor File Name") -> (w4535:string)
                n3555 = local write "standard output 2"(" ") -> ()
                n3556 = String To Path(string=w4535) -> (path=w4525:path)
                n3557 = call <vilib>:"Open_Create_Replace File.vi"("advisory dialog? (display:T)"=FALSE, "function (open:0)"=T25."create or replace", "file path"=w4525) -> ("error out"=w4538:errorcluster, "refnum"=w4537:refnum<file>)  [unwired: 5 in, 2 out]
                n3558 = Set File Position(refnum=w4537, from (0:start)=w4528, error in=w4538) -> (refnum out=w4518:refnum<file>, error out=w4517:errorcluster)  [unwired: 1 in]
                n3559 = Write to Binary File(file (use dialog)=w4518, data=" ", error in=w4517, 5:FALSE ("prepend array or string size? (T)")) -> (refnum out=w4529:refnum<file>, error out=w4530:errorcluster)  [unwired: 2 in, 1 out]
                n3560 = Set File Position(offset (in bytes) (0)=w4528, refnum=w4529, error in=w4530) -> (refnum out=w4521:refnum<file>, error out=w4520:errorcluster)  [unwired: 1 in]
                n3561 = Write to Binary File(file (use dialog)=w4521, data=w4526, error in=w4520, 5:FALSE ("prepend array or string size? (T)")) -> (error out=w4524:errorcluster)  [unwired: 2 in, 2 out]
                n3562 = flat-sequence {
                  tunnel: w4525 -> [w4540]
                  tunnel: w4524 -> [_]
                  frame #0 {
                    n3563 = call <vilib>:"Read Characters From File.vi"("file path (dialog if empty)"=w4540) -> ("character string"=→"Sensor Health JSON string":string)  [unwired: 5 in, 3 out]
                  }
                }
                "SinglePoint  2" <- w4526
              }
              frame #1 {
              }
              frame #2 {
                (unwired) "\"Stored\": true" ("string")
                n3564 = call <vilib>:"System Exec.vi"("run minimized? (F)"=TRUE, "wait until completion? (T)"=TRUE, "working directory"=path "C:/LAB-IQ-NXT", "command line"="C:\\LAB-IQ-NXT\\JPostH.bat") -> ("standard error"=→"Respose From Server 2":string, "standard output"=w4545:string)  [unwired: 4 in, 2 out]
                "standard output 2" <- w4545
                n3565 = Match Pattern(string=w4545, regular expression="JSONH Check String") -> (match substring=w4543:string, offset past match=w4542:i32)  [unwired: 1 in, 2 out]
                n3566 = Equal?(x=w4543, y="JSONH Check String") -> (x = y?=→"Upload \nConfirmed 2":bool)
              }
            }
            n3567 = Divide(x=w4385, y=3600.0 ("f")) -> (x/y=w4378:dbl)
            n3568 = local read "run time"() -> (w4435:string[])
            n3569 = Round To Nearest(number=w4378) -> (nearest integer value=w4377:dbl)
            n3570 = Number To Decimal String(number=w4377) -> (decimal integer string=w4376:string)  [unwired: 1 in]
            n3571 = Index Array(array="Sensor Information", index (col) #1=0 ("disabled index (col)"), index (col) #2=1 ("index (col)"), index (col) #3=2 ("index (col)"), index (col) #4=3 ("index (col)")) -> (element #1=→"Sensor name":string[], element #2=→"model num":string[], element #3=→"run time":string[], element #4=→"state":string[])  [unwired: 4 in]
            n3572 = Insert Into Array(array=w4435, index=1, new element #1=w4376, new element #2=w4376, new element #3=w4376, new element #4=w4376, new element #5=w4376, new element #6=w4376) -> (w4400:string[])
            "run" <- w4400
            n3573 = local read "out"() -> (w4382:string[])
            n3574 = local read "Sensor Information"() -> (w4402:string[][])
            n3575 = Replace Array Subset(array=w4402, new element #1=w4400, index (col) #1=2 ("disabled index (col)"), new element #2=w4382, index (col) #2=3 ("index (col)")) -> (w4401:string[][])  [unwired: 2 in]
            n3576 = local write "Sensor Information"(w4401) -> ()
          }
        }
        n3577 = case shown="True" w4349 {
          frame False {
          }
          frame True {
            n3578 = Equal?(x="FLAG", y=0.0) -> (x = y?=w4366:bool)
            n3579 = case shown="False" w4366 {
              frame False {
                n3580 = Get Date/Time In Seconds() -> (seconds since 1Jan1904=w4372:timestamp)
                n3581 = local read "START 2"() -> (w4370:dbl)
                n3582 = To Double Precision Float(number=w4372) -> (double precision float=w4371:dbl)
                n3583 = Subtract(x=w4371, y=w4370) -> (x-y=→"SENSOR TIME  2":dbl)
              }
              frame True {
                n3584 = Get Date/Time In Seconds() -> (seconds since 1Jan1904=w4374:timestamp)
                n3585 = To Double Precision Float(number=w4374) -> (double precision float=→"START 2":dbl)
                n3586 = local write "FLAG"(100.0 ("FLAG")) -> ()
              }
            }
          }
        }
        n3587 = disable-structure shown="Disabled" {
          disable-tunnel: w4352 -> [w4361 _]
          disable-tunnel: [w4360 _] -> w4351
          frame Disabled {
            n3588 = local read "Json St Flg"() -> (w4359:bool)
            n3589 = case shown="True" w4359 {
              tunnel: w4361 -> [w4362 w4364]
              tunnel: [w4362 w4363] -> w4360
              frame False {
              }
              frame True {
                n3590 = Increment(x=w4364) -> (x+1=w4363:dbl)
                "T cycle" <- w4363
                n3591 = local write "Json St Flg"(FALSE ("Json St Flg")) -> ()
              }
            }
          }
          frame Enabled {
          }
        }
        n3592 = local read "Quit"() -> (w4346:bool)
      }
    }
    frame Enabled {
    }
  }
  n3593 = stacked-sequence {
    tunnel: [w4744] -> w38
    frame #0 {
      w4744 = FALSE ("Upload \nConfirmed")
      n3594 = local write "Upload \nConfirmed"(w4744) -> ()
      n3595 = local write "St Str"("") -> ()
    }
  }
  n3596 = disable-structure shown="Disabled" {
    disable-tunnel: w38 -> [w4745 _]
